vi "TestRun.vi"() -> ()   [LabVIEW 2017]
uses:
  HEKAdat.lvclass
panel:
  in  "HEKAdat.lvclass IN":refnum<class "HEKAdat.lvclass">
  out "HEKAdat.lvclass OUT":refnum<class "HEKAdat.lvclass">
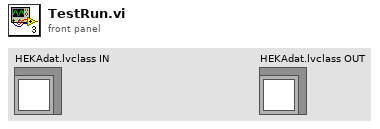
[diagram p1: front panel]
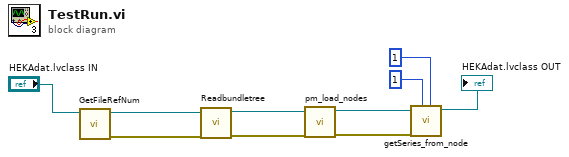
[diagram p0: block diagram]
diagram:
  n1 = call "GetFileRefNum.vi"("HEKAdat.lvclass IN"="HEKAdat.lvclass IN") -> ("Error OUT"=w9:errorcluster, "HEKAdat.lvclass OUT"=w10:refnum<class "HEKAdat.lvclass">)  [unwired: 9 in]
  n2 = call "Readbundletree.vi"("Error IN"=w9, "HEKAdat.lvclass IN"=w10) -> ("Error OUT"=w7:errorcluster, "HEKAdat.lvclass OUT"=w6:refnum<class "HEKAdat.lvclass">)  [unwired: 8 in]
  n3 = call "pm_load_nodes.vi"("Error IN"=w7, "HEKAdat.lvclass IN"=w6) -> ("Error OUT"=w5:errorcluster, "HEKAdat.lvclass OUT"=w4:refnum<class "HEKAdat.lvclass">)  [unwired: 8 in]
  n4 = call "getSeries_from_node.vi"("Series Num"=1, "Group Num"=1, "Error IN"=w5, "HEKAdat.lvclass IN"=w4) -> ("HEKAdat.lvclass OUT"=→"HEKAdat.lvclass OUT":refnum<class "HEKAdat.lvclass">)  [unwired: 5 in, 2 out]
